vi "Write FIB reheat file.vi"(8 "Reheat Parameters":T1={"Filament I (A)"=3.0, "Reheat time (s)"=45.0, "Emission (uA)"=2.2, "Calculate V/I slope"=TRUE, "Pre-calc delay (min)"=5.0, "Disable Reheat Retries"=FALSE, "Restore Voltages"=TRUE} {"Pre-calc delay (min)" format="%.2f"; "Emission (uA)" format="%.1f"; "Filament I (A)" format="%.2f"; "Reheat time (s)" format="%.1f"}, 9 "Start":bool=TRUE, 11 "Reheat file path":path=path "C:/Program Files (x86)/FEI Company/BDS/Reheat") -> ()   [LabVIEW 2018]
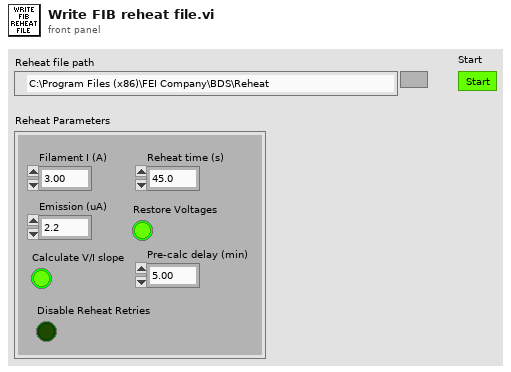
[diagram p1: front panel]
types:
  T1 = cluster{"Filament I (A)":sgl, "Reheat time (s)":sgl, "Emission (uA)":sgl, "Calculate V/I slope":bool, "Pre-calc delay (min)":sgl, "Disable Reheat Retries":bool, "Restore Voltages":bool}
  T2 = enum16{"open", "replace", "create", "open or create", "replace or create", "replace or create with confirmation"}
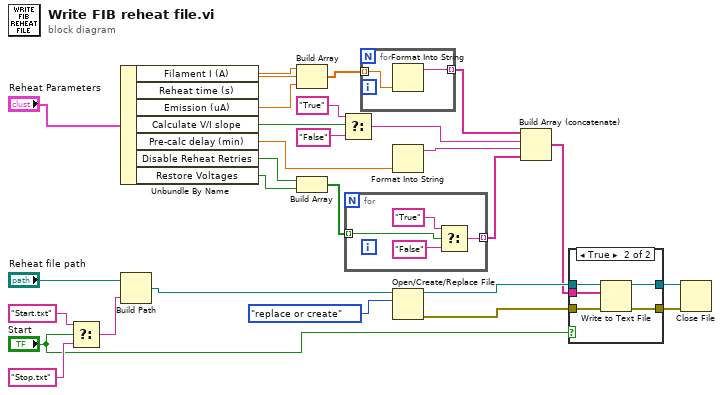
[diagram p0: block diagram]
diagram:
  n1 = Select(t="Start.txt", s="Start", f="Stop.txt") -> (s? t:f=w9:string)
  n2 = Unbundle By Name("Reheat Parameters") -> ("Filament I (A)"=w27:sgl, "Reheat time (s)"=w26:sgl, "Emission (uA)"=w25:sgl, "Calculate V/I slope"=w4:bool, "Pre-calc delay (min)"=w23:sgl, "Disable Reheat Retries"=w22:bool, "Restore Voltages"=w21:bool)
  n3 = Build Path(base path="Reheat file path", name or relative path=w9) -> (appended path=w8:path)
  n4 = Build Array(w27, w26, w25) -> (w24:sgl[])
  n5 = Build Array(w22, w21) -> (w20:bool[])
  n6 = Select(t="True" ("resulting string"), s=w4, f="False" ("resulting string")) -> (s? t:f=w1:string)
  n7 = for {
    tunnel: w20 -> [w29] mode=indexing
    tunnel: [w30] -> w5 mode=indexing
    n8 = Select(t="True" ("resulting string"), s=w29, f="False" ("resulting string")) -> (s? t:f=w30:string)
  }
  n9 = for {
    tunnel: w24 -> [w33] mode=indexing
    tunnel: [w34] -> w19 mode=indexing
    n10 = Format Into String(w33) -> (resulting string=w34:string)  [unwired: 3 in, 1 out]
  }
  n11 = Format Into String(w23) -> (resulting string=w6:string)  [unwired: 3 in, 1 out]
  n12 = Open/Create/Replace File(file path (use dialog)=w8, operation (0:open)=T2."replace or create") -> (refnum out=w16:refnum<file>, error out=w15:errorcluster)  [unwired: 1 in, 4 out]
  n13 = Build Array (concatenate)(w19, w1, w6, w5) -> (w13:string[])
  n14 = case shown="True" "Start" {
    tunnel: [w36 w41] -> w18
    tunnel: [w35 w40] -> w17
    tunnel: w16 -> [w36 w39]
    tunnel: w15 -> [w35 w38]
    tunnel: w13 -> [_ w37]
    frame False {
    }
    frame True {
      n15 = Write to Text File(file (use dialog)=w39, text=w37, error in=w38) -> (refnum out=w41:refnum<file>, error out=w40:errorcluster)  [unwired: 2 out]
    }
  }
  n16 = Close File(refnum=w18, error in=w17) -> ()  [unwired: 2 out]
